vi "AcqsitionSettingsCamera.vi"() -> ()   [LabVIEW 2019]
uses:
  <vilib>/userDefined/High Color/IMAQdx.ctl
  <vilib>/vision/driver/IMAQdx.llb/IMAQdx Camera Control Mode.ctl
  <vilib>/vision/driver/IMAQdx.llb/IMAQdx Acquisition Mode.ctl
  <vilib>/vision/driver/IMAQdx.llb/IMAQdx Buffer Number Mode.ctl
  <vilib>/vision/driver/NI_Vision_Acquisition_Software.lvlib
panel:
  out "Time 2":dbl
  out "error out 2":errorcluster
  out "Image 2":T1(plugin-control)
  in  "ImageName 2":string="name1"
  in  "Camera 2":T2="cam1"
  out "error out":errorcluster
  out "Time":dbl
  out "Image":T1(plugin-control)
  in  "Camera Control Mode":T3
  in  "Camera":T2="cam1"
  in  "ImageName":string="name1"
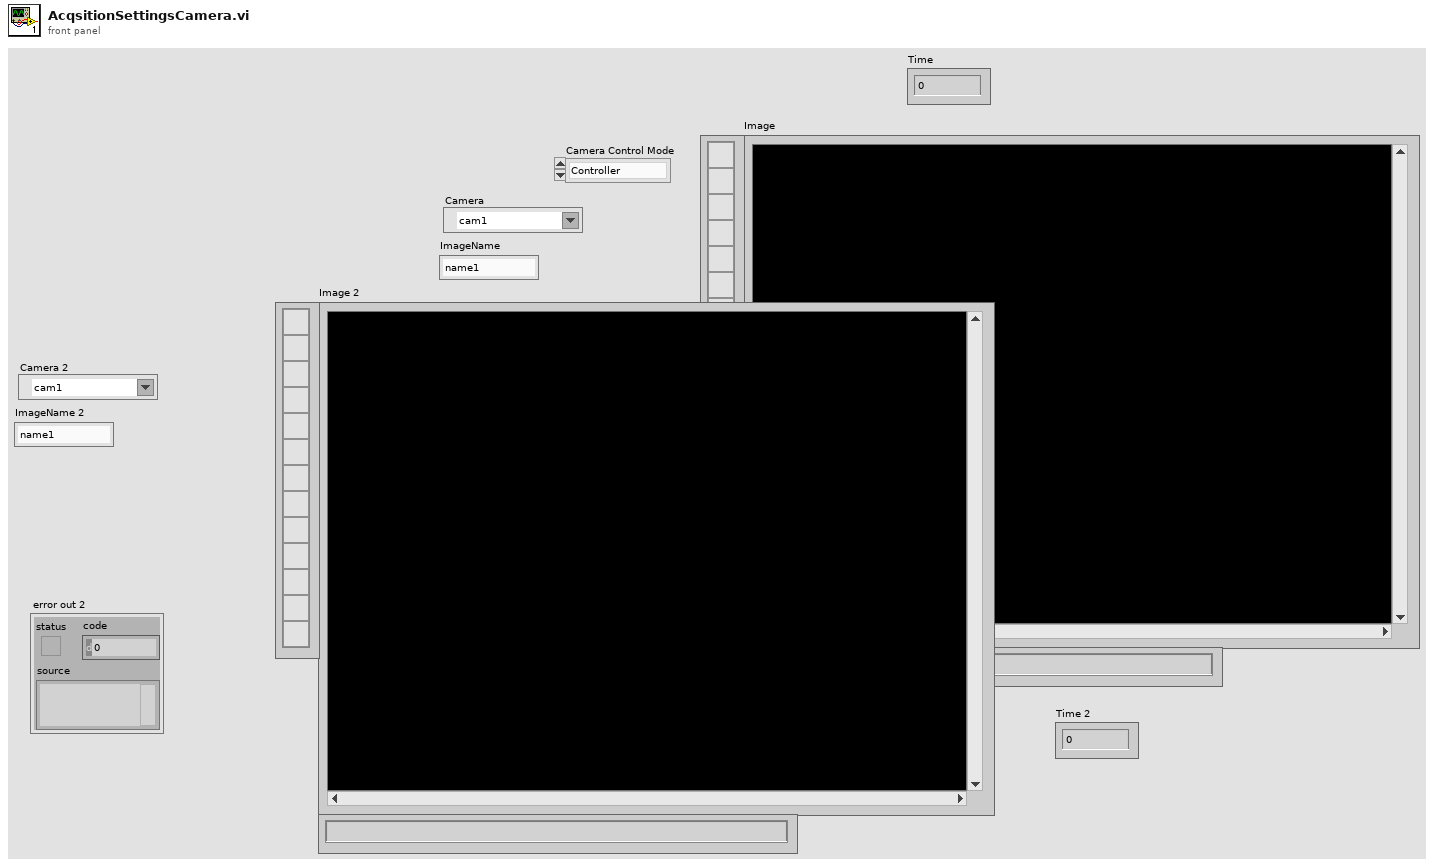
[diagram p1: front panel]
types:
  T1 = typedef "IMAQ Image.ctl" = refnum<image>
  T2 = typedef "IMAQdx.ctl" = refnum<k21>
  T3 = typedef "NI_Vision_Acquisition_Software.lvlib/IMAQdx Camera Control Mode.ctl" = enum32{"Controller", "Listener"}
  T4 = typedef "NI_Vision_Acquisition_Software.lvlib/IMAQdx Acquisition Mode.ctl" = enum32{"One Shot", "Continuous"}
  T5 = typedef "NI_Vision_Acquisition_Software.lvlib/IMAQdx Buffer Number Mode.ctl" = enum32{"Next", "Last", "Buffer Number", "Every", "Last New"}
  T6 = typedef "Image Type" = u32
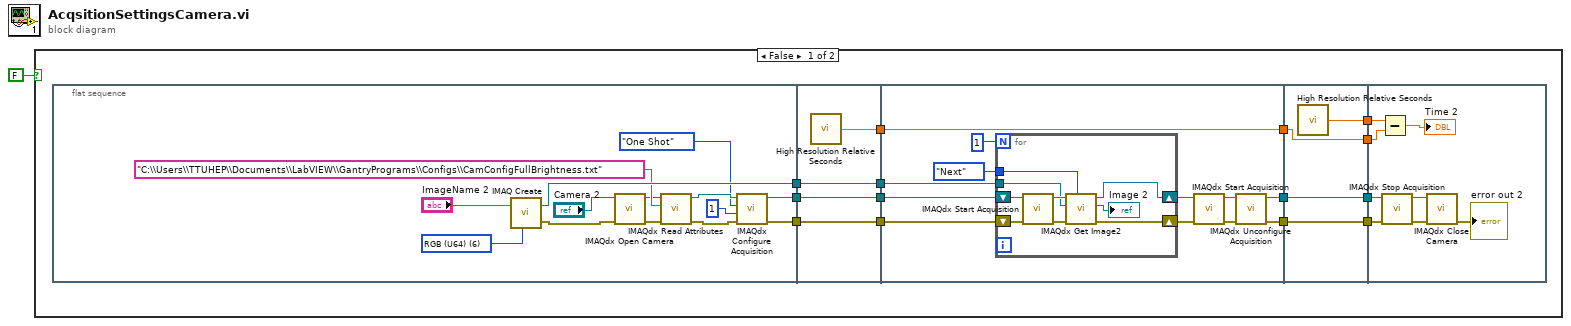
[diagram p0: block diagram]
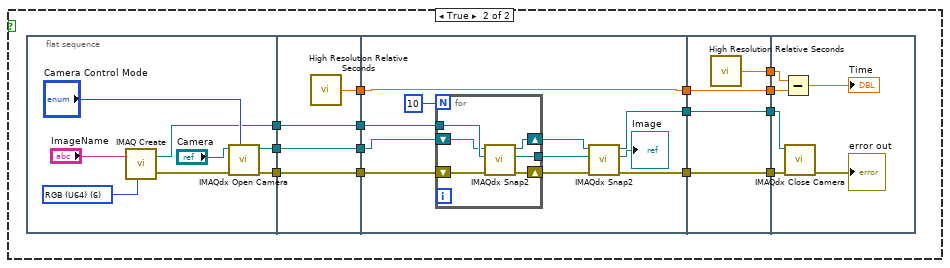
[diagram p2: hidden frame]
diagram:
  n1 = case shown="False" FALSE {
    frame False {
      n2 = flat-sequence {
        tunnel: [w21] -> w15
        tunnel: [w25] -> w14
        tunnel: [w16] -> w13
        tunnel: w15 -> [w33]
        tunnel: [w33] -> w12
        tunnel: [w32] -> w11
        tunnel: w14 -> [w32]
        tunnel: w13 -> [w31]
        tunnel: [w31] -> w10
        tunnel: [w30] -> w9
        tunnel: w12 -> [w45]
        tunnel: w11 -> [w39]
        tunnel: w10 -> [w44]
        tunnel: [w35] -> w8
        tunnel: [w34] -> w7
        tunnel: w9 -> [w42]
        tunnel: [w42] -> w6
        tunnel: w8 -> [w58]
        tunnel: [w58] -> w5
        tunnel: [w57] -> w4
        tunnel: w7 -> [w57]
        tunnel: [w56] -> w3
        tunnel: w6 -> [w55]
        tunnel: [w55] -> w2
        tunnel: w5 -> [w62]
        tunnel: w4 -> [w63]
        tunnel: w3 -> [w66]
        tunnel: w2 -> [w65]
        frame #0 {
          w26 = T6 6 items=["Grayscale (U8)", "Grayscale (I16)", "Grayscale (SGL)", "Complex (CSG)", "RGB (U32)", "HSL (U32)", "RGB (U64)", "Grayscale (U16)"] ("Image Type")
          n3 = call "IMAQ Create"("Image Name"="ImageName 2", "Image Type"=w26) -> ("New Image"=w25:T1, "error out"=w27:errorcluster)  [unwired: 3 in]
          n4 = call <vilib>:"IMAQdx Open Camera.vi"("error in"=w27, "Session In"="Camera 2") -> ("error out"=w18:errorcluster, "Session Out"=w23:T2)  [unwired: 8 in]
          n5 = call <vilib>:"IMAQdx Read Attributes.vi"("error in"=w18, "Filename"="C:\\Users\\TTUHEP\\Documents\\LabVIEW\\GantryPrograms\\Configs\\CamConfigFullBrightness.txt", "Session In"=w23) -> ("error out"=w17:errorcluster, "Session Out"=w22:T2)  [unwired: 7 in]
          n6 = call <vilib>:"IMAQdx Configure Acquisition.vi"("error in"=w17, "Number of Buffers"=u32 1, "Continuous?"=IMAQdx_Acquisition_Mode."One Shot", "Session In"=w22) -> ("error out"=w16:errorcluster, "Session Out"=w21:T2)  [unwired: 6 in]
        }
        frame #1 {
          n7 = call <vilib>:"High Resolution Relative Seconds.vi"() -> ("relative seconds"=w30:dbl)
        }
        frame #2 {
          n8 = for {
            N: 1 -> [_]
            tunnel: w39 -> [w50]
            shift-right: [w46] -> w41
            shift-left: w45 -> [w54]
            shift-right: [w48] -> w40
            shift-left: w44 -> [w53]
            tunnel: IMAQdx_Buffer_Number_Mode."Next" ("Buffer Number Mode (Next)") -> [w52]
            n9 = call <vilib>:"IMAQdx Start Acquisition.vi"("error in"=w53, "Session In"=w54) -> ("error out"=w49:errorcluster, "Session Out"=w51:T2)  [unwired: 8 in]
            n10 = call <vilib>:"IMAQdx Get Image2.vi"("Buffer Number Mode (Next)"=w52, "error in"=w49, "Image In"=w50, "Session In"=w51) -> ("error out"=w48:errorcluster, "Image Out"=→"Image 2":T1, "Session Out"=w46:T2)  [unwired: 4 in, 1 out]
          }
          n11 = call <vilib>:"IMAQdx Start Acquisition.vi"("error in"=w40, "Session In"=w41) -> ("error out"=w36:errorcluster, "Session Out"=w37:T2)  [unwired: 8 in]
          n12 = call <vilib>:"IMAQdx Unconfigure Acquisition.vi"("error in"=w36, "Session In"=w37) -> ("error out"=w35:errorcluster, "Session Out"=w34:T2)  [unwired: 8 in]
        }
        frame #3 {
          n13 = call <vilib>:"High Resolution Relative Seconds.vi"() -> ("relative seconds"=w56:dbl)
        }
        frame #4 {
          n14 = Subtract(x=w66, y=w65) -> (x-y=→"Time 2":dbl)
          n15 = call <vilib>:"IMAQdx Stop Acquisition.vi"("error in"=w62, "Session In"=w63) -> ("error out"=w60:errorcluster, "Session Out"=w61:T2)  [unwired: 8 in]
          n16 = call <vilib>:"IMAQdx Close Camera.vi"("error in"=w60, "Session In"=w61) -> ("error out"=→"error out 2":errorcluster)  [unwired: 9 in]
        }
      }
    }
    frame True {
      n17 = flat-sequence {
        tunnel: [w84] -> w80
        tunnel: [w82] -> w79
        tunnel: [w81] -> w78
        tunnel: w80 -> [w92]
        tunnel: [w92] -> w77
        tunnel: [w91] -> w76
        tunnel: w79 -> [w91]
        tunnel: w78 -> [w90]
        tunnel: [w90] -> w75
        tunnel: [w89] -> w74
        tunnel: w77 -> [w100]
        tunnel: w76 -> [w101]
        tunnel: w75 -> [w99]
        tunnel: [w103] -> w73
        tunnel: [w102] -> w72
        tunnel: w74 -> [w93]
        tunnel: [w93] -> w71
        tunnel: w73 -> [w113]
        tunnel: [w113] -> w70
        tunnel: [w112] -> w69
        tunnel: w72 -> [w112]
        tunnel: [w111] -> w68
        tunnel: w71 -> [w110]
        tunnel: [w110] -> w67
        tunnel: w70 -> [w119]
        tunnel: w69 -> [w118]
        tunnel: w68 -> [w117]
        tunnel: w67 -> [w116]
        frame #0 {
          w85 = T6 6 items=["Grayscale (U8)", "Grayscale (I16)", "Grayscale (SGL)", "Complex (CSG)", "RGB (U32)", "HSL (U32)", "RGB (U64)", "Grayscale (U16)"] ("Image Type")
          n18 = call "IMAQ Create"("Image Name"="ImageName", "Image Type"=w85) -> ("New Image"=w82:T1, "error out"=w86:errorcluster)  [unwired: 3 in]
          n19 = call <vilib>:"IMAQdx Open Camera.vi"("Camera Control Mode"="Camera Control Mode", "error in"=w86, "Session In"="Camera") -> ("error out"=w81:errorcluster, "Session Out"=w84:T2)  [unwired: 7 in]
        }
        frame #1 {
          n20 = call <vilib>:"High Resolution Relative Seconds.vi"() -> ("relative seconds"=w89:dbl)
        }
        frame #2 {
          n21 = for {
            N: 10 -> [_]
            tunnel: w101 -> [w109]
            shift-right: [w105] -> w97
            shift-left: w100 -> [w108]
            shift-right: [w106] -> w98
            shift-left: w99 -> [w107]
            tunnel: [w104] -> w94
            n22 = call <vilib>:"IMAQdx Snap2.vi"("error in"=w107, "Image In"=w109, "Session In"=w108) -> ("error out"=w106:errorcluster, "Image Out"=w104:T1, "Session Out"=w105:T2)  [unwired: 6 in]
          }
          n23 = call <vilib>:"IMAQdx Snap2.vi"("error in"=w98, "Image In"=w94, "Session In"=w97) -> ("error out"=w103:errorcluster, "Image Out"=→"Image":T1, "Session Out"=w102:T2)  [unwired: 6 in]
        }
        frame #3 {
          n24 = call <vilib>:"High Resolution Relative Seconds.vi"() -> ("relative seconds"=w111:dbl)
        }
        frame #4 {
          n25 = Subtract(x=w117, y=w116) -> (x-y=→"Time":dbl)
          n26 = call <vilib>:"IMAQdx Close Camera.vi"("error in"=w119, "Session In"=w118) -> ("error out"=→"error out":errorcluster)  [unwired: 9 in]
        }
      }
    }
  }
